vi "set_config_cluster.vi"(8 "error in (no error)":errorcluster, 10 "config cluster variant":variant, 11 "LightSourceAN191011Chameleon in":refnum<class "LightSourceAN191011Chameleon.lvclass">) -> (0 "error out":errorcluster, 3 "LightSourceAN191011Chameleon out":refnum<class "LightSourceAN191011Chameleon.lvclass">)   [LabVIEW 2011, in "LightSourceAN191011Chameleon.lvclass"]
uses:
  LightSourceAN191011Chameleon.lvclass
  LightSourceAN191011Chameleon.lvclass/LightSourceAN191011Chameleon.ctl
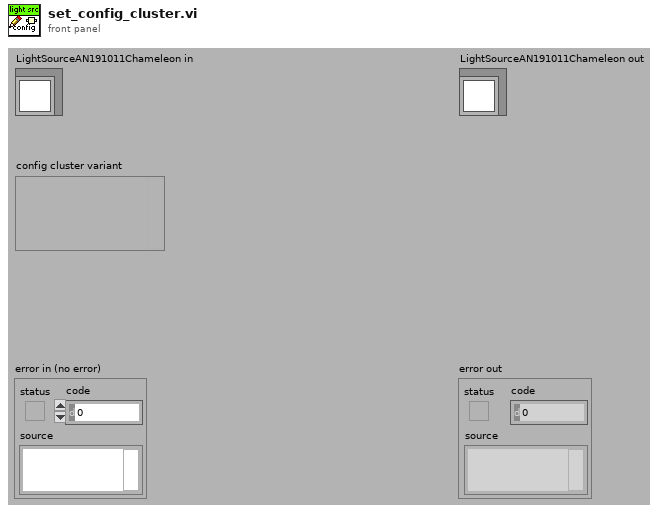
[diagram p1: front panel]
types:
  T1 = typedef "LightSourceAN191011Chameleon.lvclass/config_data.ctl" = cluster{"communication settings":cluster{"comm port":string, "data bits":u16, "parity":enum16{"None", "Odd", "Even", "Mark", "Space"}, "baud rate":u32, "delay before read":u32, "stop bits":u16}, "OME":cluster{"LSID":T2}, "laser settings":cluster{"start wavelength":dbl[unit]}}
  T2 = typedef "LSID_cluster.ctl" = cluster{"identifier":string, "revision":i32}
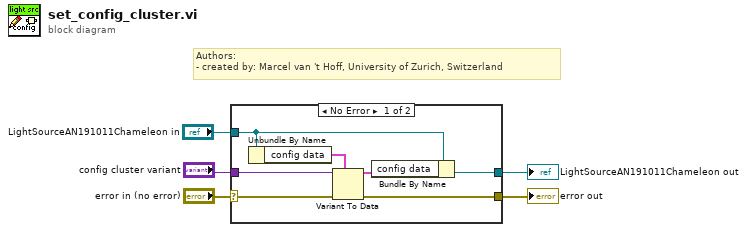
[diagram p0: block diagram]
diagram:
  # "Authors: \n- created by: Marcel van 't Hoff, University of Zurich, Switzerland"
  n1 = case shown="No Error" "error in (no error)" {
    selector: "error in (no error)" -> [w10 w14]
    tunnel: [w6 w14] -> w4
    tunnel: [w7 w13] -> w3
    tunnel: "LightSourceAN191011Chameleon in" -> [w9 w13]
    tunnel: "config cluster variant" -> [w12 _]
    frame No Error {
      n2 = Unbundle By Name(w9) -> ("config data"=w11:T1)
      n3 = Variant To Data(error in=w10, type=w11, Variant=w12) -> (data=w8:T1, error out=w6:errorcluster)
      n4 = Bundle By Name(cluster=w9, "config data"=w8) -> (w7:refnum<class "LightSourceAN191011Chameleon.lvclass">)
    }
    frame Error {
    }
  }
  "error out" <- w4
  "LightSourceAN191011Chameleon out" <- w3
